vi "Acquisition.vi"() -> ()   [LabVIEW 2012]
uses:
  Type/_Run State.ctl
  Type/_File Type.ctl
  Type/_RT Command.ctl
  Type/_Data Operation.ctl
  Type/_Run Module.ctl
  Configuration/_Global Configuration.vi
  <vilib>/Utility/config.llb/Read Key (Path).vi
  <vilib>/Utility/config.llb/Read Key (String).vi
  <vilib>/Utility/config.llb/Write Key (Path).vi
  <vilib>/Utility/config.llb/Write Key (String).vi
  <vilib>/Utility/file.llb/Read From Spreadsheet File (string).vi
  <vilib>/Utility/config.llb/NI_LVConfig.lvlib
  <vilib>/Utility/miscctls.llb/LVRectTypeDef.ctl
panel:
  in  "Equilibration Time":u32
  in  "Editor":bool
  out "# of Samp":i32=1 caption="# of Samples"
  in  "Sample Description":string
  in  "Sync Mode":enum32{"Manual", "LC Sync"}(radio)
  in  "Data Folder":path
  in  "Save":bool
  in  "Load":bool
  in  "Insert":bool
  in  "Delete":bool
  in  "Import":bool
  in  "Export":bool
  in  "Sample List":i32(listbox)
  in  "Run":bool
  in  "Cancel":bool
  in  "List File":path
  out "Run Time":i32=1 caption="Run Time (ms)"
  in  "Current Sample":i32=1 min=0
  in  "Method File":path
  # "(mS)"
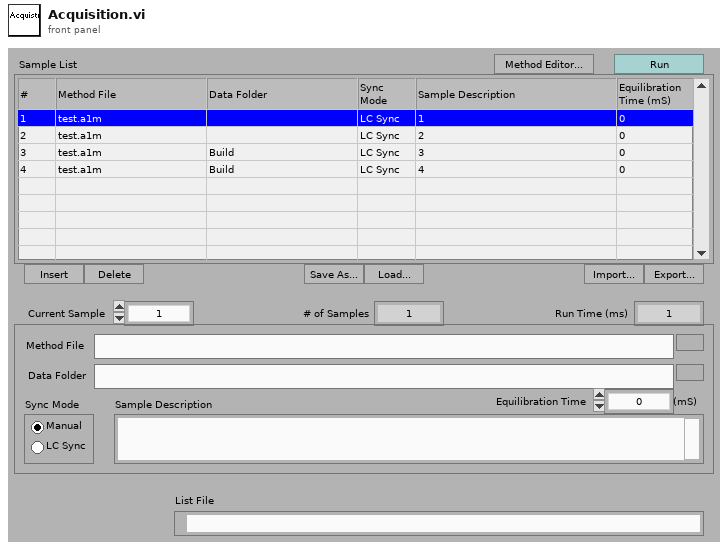
[diagram p1: front panel]
types:
  T1 = typedef "_Run State.ctl" = enum16{"Init", "Update", "Start", "End", "Error"}
  T2 = typedef "_File Type.ctl" = enum16{"Configuration", "Old Configuration", "Calibration", "Resolution", "Diagnostic Method", "Old Method", "Acq Method", "Samp List"}
  T3 = typedef "LVRectTypeDef.ctl" = cluster{"Left":i16, "Top":i16, "Right":i16, "Bottom":i16}
  T4 = typedef "_RT Command.ctl" = enum16{"Start", "Stop", "Runtime Update", "Get Data", "Get Info", "Get Status", "Get Param", "Get Config", "Get Table", "Read ADC", "Set Oscillator", "Update Config", "Update Table", "Set All Pol", "Set Pol and DC", "Set Max Mass", "Toggle RP", "Toggle EL", "Set PIC", "Initialize Turbo", "Send Turbo Comm", "Close Turbo", "P1", "P2", "P3", "Send Serial", "Set LC Out", "Get LC In", "Read VAC", "Test Table", "Toggle Power", "Get Startup", "Set Startup", "Get ADC Table", "Set ADC Table", "Get Brief Status", "Get Detail Status", "Auxiliary Update", "Set CC Logics", "Set CC Input Logics", "Ignore Error"}
  T5 = typedef "_Data Operation.ctl" = enum8{"Initialize", "Get Data", "Set Data", "Close"}
  T6 = enum32{"Bad", "Idle", "Run top level", "Running"}
  T7 = enum32{"existing file", "new file", "new or existing file", "existing dir", "new dir", "new or existing dir", "existing file (use LLBs)", "new file (use LLBs)", "new or existing file (use LLBs)", "new or existing file or directory (use LLBs)"}
  T8 = typedef "NI_LVConfig.lvlib/Config Data RefNum.ctl" = refnum<k1>
  T9 = cluster{"Update":bool, "Running":bool, "List File":path, "Sample List":string[][]}
  T10 = typedef "_Run Module.ctl" = u16
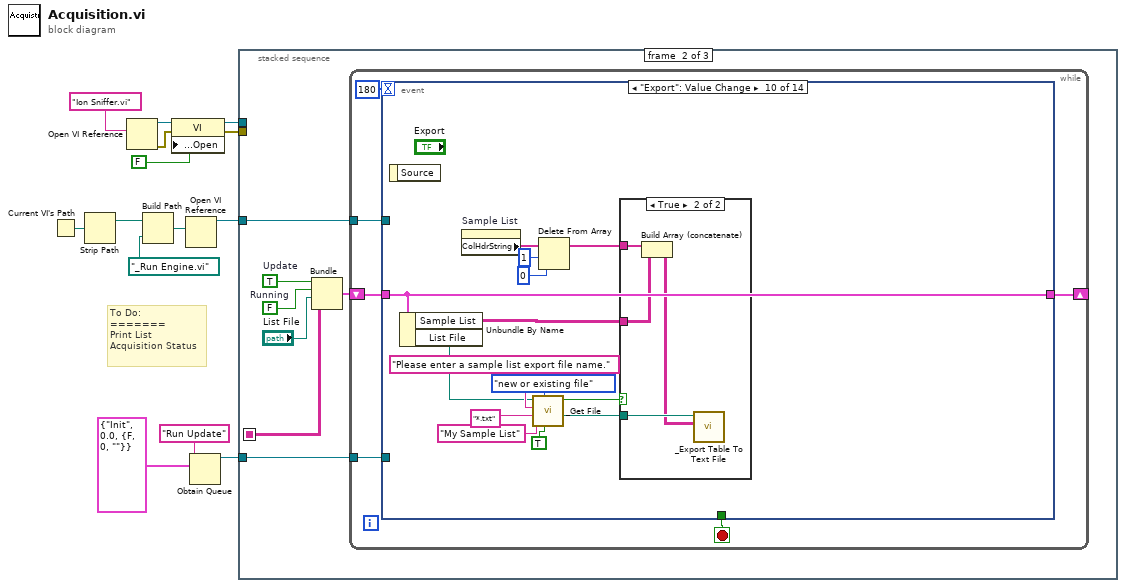
[diagram p0: block diagram]
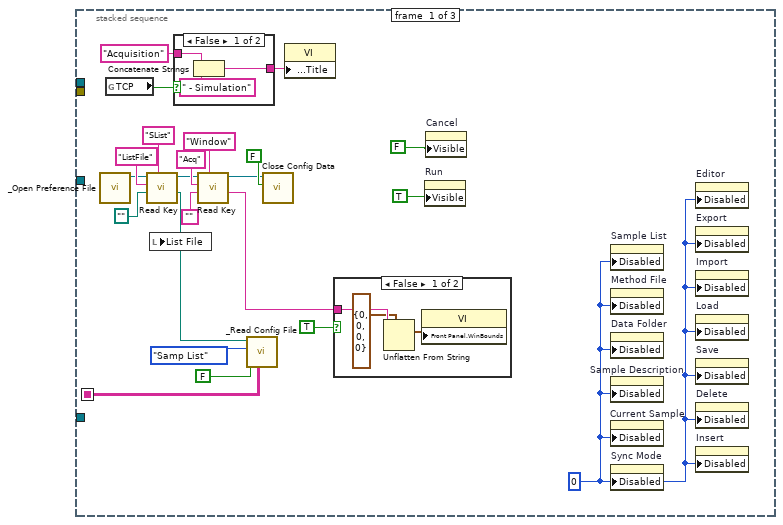
[diagram p2: hidden frame]
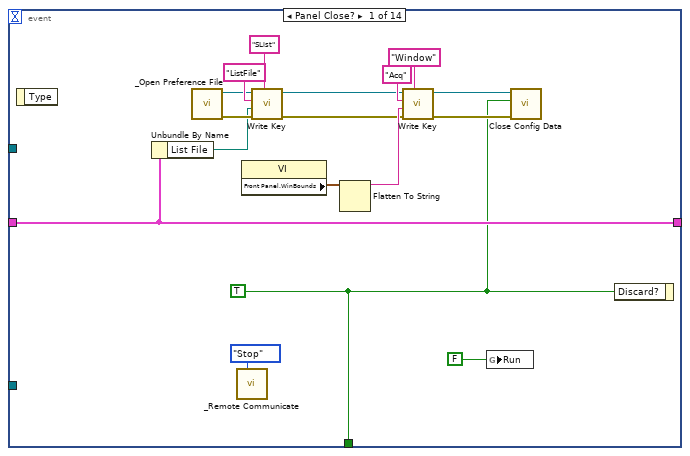
[diagram p5: hidden frame]
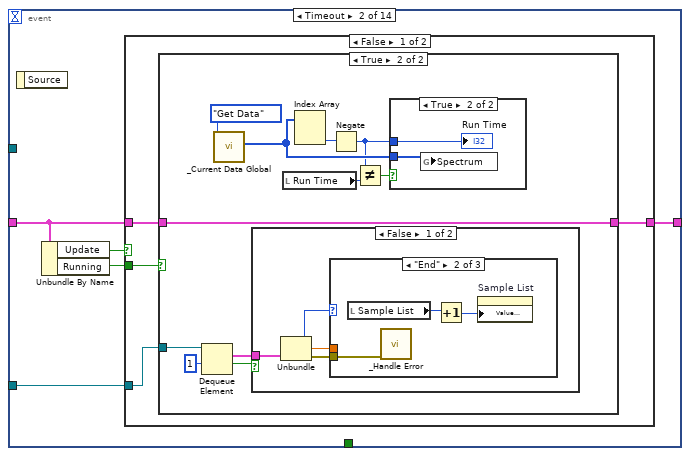
[diagram p6: hidden frame]
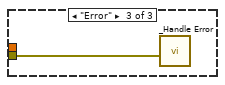
[diagram p10: hidden frame]
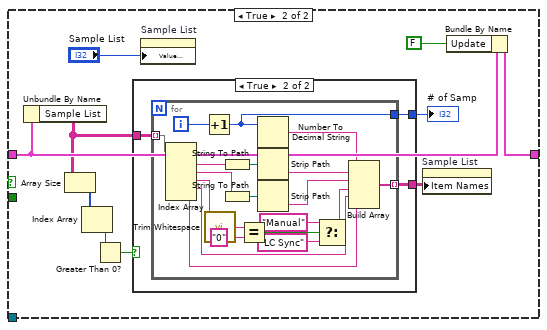
[diagram p12: hidden frame]
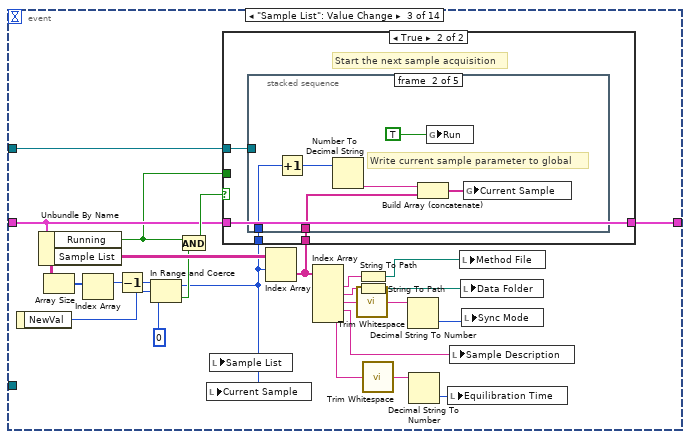
[diagram p14: hidden frame]
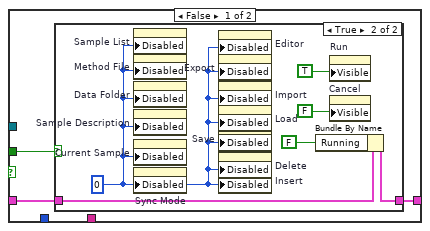
[diagram p15: hidden frame]
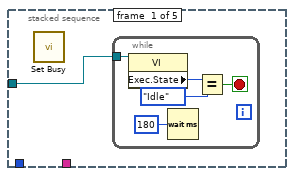
[diagram p17: hidden frame]
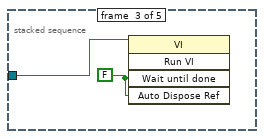
[diagram p18: hidden frame]
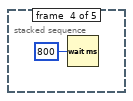
[diagram p19: hidden frame]
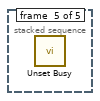
[diagram p20: hidden frame]
diagram:
  # "To Do:\n=======\nPrint List\nAcquisition Status"
  n1 = Current VI's Path() -> (path=w11:path)
  n2 = Strip Path(path=w11) -> (stripped path=w7:path)  [unwired: 1 out]
  n3 = Open VI Reference(vi path="Ion Sniffer.vi") -> (vi reference=w5:refnum<vi>, error out=w4:errorcluster)  [unwired: 1 in, 4 out]
  n4 = Build Path(base path=w7, name or relative path=path "_Run Engine.vi") -> (appended path=w9:path)
  n5 = property class="VI"(reference=w5, error in=w4, "Front Panel Window:Open"=FALSE) -> (reference out=w2:refnum<vi>, error out=w1:errorcluster)
  n6 = Open VI Reference(vi path=w9) -> (vi reference=w8:refnum<vi>)  [unwired: 1 in, 5 out]
  n7 = Obtain Queue(name (unnamed)="Run Update", element data type=cluster{T1, dbl, "error out":errorcluster} {enum."Init", 0.0, "error out"={"status"=FALSE, "code"=0, "source"=""}}) -> (queue out=w12:refnum<queue>)  [unwired: 3 in, 2 out]
  n8 = stacked-sequence {
    seq-local: [w17 _ _] -> [_ w44 _]
    tunnel: w12 -> [_ w50 w346]
    tunnel: w8 -> [_ w49 w345]
    tunnel: w2 -> [_ _ w341]
    tunnel: w1 -> [_ _ w340]
    frame #0 {
      w16 = u8 0 ("Disabled")
      n9 = call "_Open Preference File.vi"() -> ("refnum"=w22:T8)  [unwired: 1 in, 6 out]
      n10 = global read "_Global Configuration.vi" "TCP"() -> (w34:bool)
      n11 = call-poly <vilib>:"Read Key.vi"("section"="SList", "default value"=path "", "key"="ListFile", "refnum"=w22) -> ("value"=w18:path, "refnum out"=w23:T8)  [unwired: 1 in, 5 out]
      n12 = local write "List File"(w18) -> ()
      n13 = case shown="False" w34 {
        tunnel: "Acquisition" ("string") -> [w42 w43]
        tunnel: [w40 w43] -> w35
        frame False {
          n14 = Concatenate Strings(w42, " - Simulation" ("string")) -> (w40:string)
        }
        frame True {
        }
      }
      n15 = call-poly <vilib>:"Read Key.vi"("section"="Window", "default value"="", "key"="Acq" ("section"), "refnum"=w23) -> ("value"=w25:string, "refnum out"=w21:T8)  [unwired: 2 in, 4 out]
      n16 = call "_Read Config File.vi"("advisory dialog? (display:T)"=FALSE, "File Type (config)"=_File_Type."Samp List", "start path  (Not A Path)"=w18) -> ("Sample List"=w17:string[][])  [unwired: 8 out]
      n17 = call <vilib>:"Close Config Data.vi"("write file if changed (T)"=FALSE ("write configuration file? (F)"), "refnum"=w21) -> ()  [unwired: 1 in, 9 out]
      n18 = property class="VI"("Front Panel Window:Title"=w35) -> ()  [unwired: 2 in, 2 out]
      n19 = case shown="False" TRUE {
        tunnel: w25 -> [w39 _]
        frame False {
          n20 = Unflatten From String(type=T3 {"Left"=0, "Top"=0, "Right"=0, "Bottom"=0} ("Front Panel Window:Window Bounds"), binary string=w39) -> (value=w37:T3)  [unwired: 1 in, 4 out]
          n21 = property class="VI"("Front Panel.WinBounds"=w37) -> ()  [unwired: 2 in, 2 out]
        }
        frame True {
        }
      }
      n22 = property on="Run" class="Bool"("Visible"=TRUE) -> ()  [unwired: 2 in, 2 out]
      n23 = property on="Cancel" class="Bool"("Visible"=FALSE ("Unit")) -> ()  [unwired: 2 in, 2 out]
      n24 = property on="Sample List" class="MCListbox (strict)"("Disabled"=w16) -> ()  [unwired: 2 in, 2 out]
      n25 = property on="Method File" class="Path"("Disabled"=w16) -> ()  [unwired: 2 in, 2 out]
      n26 = property on="Data Folder" class="Path"("Disabled"=w16) -> ()  [unwired: 2 in, 2 out]
      n27 = property on="Sample Description" class="Str"("Disabled"=w16) -> ()  [unwired: 2 in, 2 out]
      n28 = property on="Current Sample" class="DigNum (strict)"("Disabled"=w16) -> ()  [unwired: 2 in, 2 out]
      n29 = property on="Sync Mode" class="RadioBtnsControl (strict)"("Disabled"=w16) -> ()  [unwired: 2 in, 2 out]
      n30 = property on="Editor" class="Bool"("Disabled"=w16) -> ()  [unwired: 2 in, 2 out]
      n31 = property on="Export" class="Bool"("Disabled"=w16) -> ()  [unwired: 2 in, 2 out]
      n32 = property on="Import" class="Bool"("Disabled"=w16) -> ()  [unwired: 2 in, 2 out]
      n33 = property on="Load" class="Bool"("Disabled"=w16) -> ()  [unwired: 2 in, 2 out]
      n34 = property on="Save" class="Bool"("Disabled"=w16) -> ()  [unwired: 2 in, 2 out]
      n35 = property on="Delete" class="Bool"("Disabled"=w16) -> ()  [unwired: 2 in, 2 out]
      n36 = property on="Insert" class="Bool"("Disabled"=w16) -> ()  [unwired: 2 in, 2 out]
    }
    frame #1 {
      w47 = FALSE  # Running
      w48 = TRUE  # Update
      n37 = Bundle("Update"=w48, "Running"=w47, "List File"="List File", "Sample List"=w44) -> (w46:T9)  [unwired: 1 out]
      n38 = while {
        shift-right: [w53] -> _
        shift-left: w46 -> [w55]
        tunnel: w50 -> [w52]
        tunnel: w49 -> [w51]
        stop <- w56 stop-if-true
        n39 = event shown="[9] \"Export\": Value Change" {
          selector: _ -> [_ _ _ _ _ _ _ _ _ _ _ _ _ _]
          dyn-events: _ -> [_ _ _ _ _ _ _ _ _ _ _ _ _ _]
          timeout: 180 -> [_ _ _ _ _ _ _ _ _ _ _ _ _ _]
          tunnel: [w57 _ _ _ _ _ _ _ _ _ _ _ _ _] -> w56
          tunnel: w55 -> [w68 w76 w145 w193 w209 w222 w230 w244 w252 w272 w308 w311 w325 w339]
          tunnel: [w68 w78 w144 w193 w208 w220 w228 w242 w251 w272 w310 w318 w321 w339] -> w53
          tunnel: w52 -> [_ w77 _ _ _ _ _ _ _ _ _ w320 _ _]
          tunnel: w51 -> [_ _ w146 _ _ _ _ _ _ _ _ _ w324 _]
          event Panel Close? {
            w57 = TRUE ("Discard?")
            n40 = event-data() -> ()  [unwired: 2 out]
            n41 = Unbundle By Name(w68) -> ("List File"=w67:path)
            n42 = call "_Open Preference File.vi"() -> ("error"=w70:errorcluster, "refnum"=w71:T8)  [unwired: 1 in, 5 out]
            n43 = call "_Remote Communicate.vi"("Command"=_RT_Command."Stop") -> ()  [unwired: 5 in, 4 out]
            n44 = property class="VI"() -> ("Front Panel.WinBounds"=w65:T3)  [unwired: 2 in, 2 out]
            n45 = call-poly <vilib>:"Write Key.vi"("section"="SList", "error in (no error)"=w70, "value"=w67, "key"="ListFile", "refnum"=w71) -> ("error out"=w58:errorcluster, "refnum out"=w59:T8)  [unwired: 5 out]
            n46 = Flatten To String(anything=w65) -> (data string=w64:string)  [unwired: 1 in, 4 out]
            n47 = call-poly <vilib>:"Write Key.vi"("section"="Window", "error in (no error)"=w58, "value"=w64, "key"="Acq" ("section"), "refnum"=w59) -> ("error out"=w60:errorcluster, "refnum out"=w61:T8)  [unwired: 1 in, 4 out]
            n48 = global write "_Global Configuration.vi" "Run"(FALSE ("Update")) -> ()
            n49 = call <vilib>:"Close Config Data.vi"("error in (no error)"=w60, "write file if changed (T)"=w57, "refnum"=w61) -> ()  [unwired: 9 out]
            n50 = event-data("Discard?"=w57) -> ()  [unwired: 1 in, 1 out]
          }
          event Timeout {
            n51 = event-data() -> ()  [unwired: 2 out]
            n52 = Unbundle By Name(w76) -> ("Update"=w75:bool, "Running"=w74:bool)
            n53 = case shown="False" w75 {
              tunnel: w76 -> [w80 w114]
              tunnel: [w79 w112] -> w78
              tunnel: w74 -> [w82 _]
              tunnel: w77 -> [w81 _]
              frame False {
                n54 = case shown="True" w82 {
                  tunnel: w81 -> [_ w94]
                  tunnel: w80 -> [w83 w84]
                  tunnel: [w83 w84] -> w79
                  frame False {
                  }
                  frame True {
                    n55 = Dequeue Element(queue=w94, timeout in ms (-1)=1) -> (element=w92:cluster{T1, dbl, "error out":errorcluster}, timed out?=w91:bool)  [unwired: 1 in, 2 out]
                    n56 = call "_Current Data Global.vi"("Operation"=_Data_Operation."Get Data") -> ("Latest Raw Data"=w87:i32[])  [unwired: 3 in, 3 out]
                    n57 = case shown="False" w91 {
                      tunnel: w92 -> [w100 _]
                      frame False {
                        n58 = Unbundle(w100) -> (w99:T1, w97:dbl, "error out"=w98:errorcluster)
                        n59 = case shown="\"End\"" w99 {
                          tunnel: w98 -> [_ w103 w104]
                          tunnel: w97 -> [_ _ _]
                          frame "Init", Default {
                          }
                          frame "End" {
                            n60 = local read "Sample List"() -> (w102:i32)
                            n61 = call "_Handle Error.vi"("error in (no error)"=w103) -> ()  [unwired: 2 in, 5 out]
                            n62 = Increment(x=w102) -> (x+1=w101:i32)
                            n63 = property on="Sample List" class="MCListbox (strict)"("Value (Signaling)"=w101) -> ()  [unwired: 2 in, 2 out]
                          }
                          frame "Error" {
                            n64 = call "_Handle Error.vi"("error in (no error)"=w104) -> ()  [unwired: 2 in, 5 out]
                          }
                        }
                      }
                      frame True {
                      }
                    }
                    n65 = local read "Run Time"() -> (w89:i32)
                    n66 = Index Array(array=w87) -> (element #2=w86:i32)  [unwired: 2 in, 1 out]
                    n67 = Negate(x=w86) -> (-x=w85:i32)
                    n68 = Not Equal?(x=w85, y=w89) -> (x != y?=w88:bool)
                    n69 = case shown="True" w88 {
                      tunnel: w87 -> [_ w95]
                      tunnel: w85 -> [_ w96]
                      frame False {
                      }
                      frame True {
                        n70 = global write "_Global Configuration.vi" "Spectrum"(w95) -> ()
                        "Run Time" <- w96
                      }
                    }
                  }
                }
              }
              frame True {
                n71 = Unbundle By Name(w114) -> ("Sample List"=w108:string[][])
                n72 = Array Size(array=w108) -> (size(s)=w107:i32[])
                n73 = Index Array(array=w107) -> (element=w106:i32)  [unwired: 1 in]
                n74 = Greater Than 0?(x=w106) -> (x > 0?=w105:bool)
                n75 = case shown="True" w105 {
                  tunnel: [_ w117] -> w110
                  tunnel: [_ w116] -> w109
                  tunnel: w108 -> [_ w115]
                  frame False {
                  }
                  frame True {
                    n76 = for {
                      tunnel: w115 -> [w137] mode=indexing
                      tunnel: [w135] -> w117
                      tunnel: [w120] -> w116 mode=indexing
                      i -> [w136]
                      n77 = Index Array(array=w137) -> (element #1=w134:string, element #2=w131:string, element #3=w130:string, element #4=w121:string, element #5=w118:string)  [unwired: 5 in]
                      n78 = Increment(x=w136) -> (x+1=w135:i32)
                      n79 = call <vilib>:"Trim Whitespace.vi"("string"=w130) -> ("trimmed string"=w128:string)  [unwired: 1 in]
                      n80 = String To Path(string=w134) -> (path=w133:path)
                      n81 = String To Path(string=w131) -> (path=w132:path)
                      n82 = Equal?(x=w128, y="0") -> (x = y?=w129:bool)
                      n83 = Number To Decimal String(number=w135) -> (decimal integer string=w125:string)  [unwired: 1 out]
                      n84 = Strip Path(path=w133) -> (name=w124:string)  [unwired: 1 out]
                      n85 = Strip Path(path=w132) -> (name=w123:string)  [unwired: 1 out]
                      n86 = Select(t="Manual" ("y"), s=w129, f="LC Sync" ("y")) -> (s? t:f=w122:string)
                      n87 = Build Array(w125, w124, w123, w122, w121, w118) -> (w120:string[])
                    }
                  }
                }
                "# of Samp" <- w110
                n88 = property on="Sample List" class="MCListbox (strict)"("Value (Signaling)"="Sample List") -> ()  [unwired: 2 in, 2 out]
                n89 = property on="Sample List" class="MCListbox (strict)"("Item Names"=w109) -> ()  [unwired: 2 in, 2 out]
                n90 = Bundle By Name(cluster=w114, "Update"=FALSE) -> (w112:T9)
              }
            }
          }
          event "Sample List": Value Change {
            n91 = event-data() -> ("NewVal"=w162:i32)  [unwired: 1 out]
            n92 = Unbundle By Name(w145) -> ("Running"=w143:bool, "Sample List"=w159:string[][])
            n93 = Array Size(array=w159) -> (size(s)=w157:i32[])
            n94 = Index Array(array=w157) -> (element=w158:i32)  [unwired: 1 in]
            n95 = Decrement(x=w158) -> (x-1=w160:i32)
            n96 = In Range and Coerce(upper limit=w160, x=w162, lower limit=0) -> (coerced(x)=w141:i32, In Range?=w148:bool)
            n97 = And(x=w143, y=w148) -> (x .and. y?=w147:bool)
            n98 = local write "Current Sample"(w141) -> ()
            n99 = local write "Sample List"(w141) -> ()
            n100 = Index Array(array=w159, index (row)=w141) -> (element=w142:string[])  [unwired: 1 in]
            n101 = case shown="True" w147 {
              tunnel: w146 -> [_ w176]
              tunnel: w145 -> [w165 w175]
              tunnel: [w164 w175] -> w144
              tunnel: w143 -> [w163 _]
              tunnel: w142 -> [_ w174]
              tunnel: w141 -> [_ w173]
              frame False {
                n102 = case shown="True" w163 {
                  tunnel: w165 -> [w166 w172]
                  tunnel: [w166 w171] -> w164
                  frame False {
                  }
                  frame True {
                    w170 = u8 0 ("Disabled")
                    n103 = property on="Sample List" class="MCListbox (strict)"("Disabled"=w170) -> ()  [unwired: 2 in, 2 out]
                    n104 = property on="Method File" class="Path"("Disabled"=w170) -> ()  [unwired: 2 in, 2 out]
                    n105 = property on="Data Folder" class="Path"("Disabled"=w170) -> ()  [unwired: 2 in, 2 out]
                    n106 = property on="Sample Description" class="Str"("Disabled"=w170) -> ()  [unwired: 2 in, 2 out]
                    n107 = property on="Current Sample" class="DigNum (strict)"("Disabled"=w170) -> ()  [unwired: 2 in, 2 out]
                    n108 = property on="Sync Mode" class="RadioBtnsControl (strict)"("Disabled"=w170) -> ()  [unwired: 2 in, 2 out]
                    n109 = property on="Editor" class="Bool"("Disabled"=w170) -> ()  [unwired: 2 in, 2 out]
                    n110 = property on="Export" class="Bool"("Disabled"=w170) -> ()  [unwired: 2 in, 2 out]
                    n111 = property on="Import" class="Bool"("Disabled"=w170) -> ()  [unwired: 2 in, 2 out]
                    n112 = property on="Load" class="Bool"("Disabled"=w170) -> ()  [unwired: 2 in, 2 out]
                    n113 = property on="Save" class="Bool"("Disabled"=w170) -> ()  [unwired: 2 in, 2 out]
                    n114 = property on="Delete" class="Bool"("Disabled"=w170) -> ()  [unwired: 2 in, 2 out]
                    n115 = property on="Insert" class="Bool"("Disabled"=w170) -> ()  [unwired: 2 in, 2 out]
                    n116 = Bundle By Name(cluster=w172, "Running"=FALSE) -> (w171:T9)
                    n117 = property on="Run" class="Bool"("Visible"=TRUE) -> ()  [unwired: 2 in, 2 out]
                    n118 = property on="Cancel" class="Bool"("Visible"=FALSE) -> ()  [unwired: 2 in, 2 out]
                  }
                }
              }
              frame True {
                # "Start the next sample acquisition"
                n119 = stacked-sequence {
                  tunnel: w176 -> [w177 _ w189 _ _]
                  tunnel: w174 -> [_ w187 _ _ _]
                  tunnel: w173 -> [_ w184 _ _ _]
                  frame #0 {
                    n120 = call <vilib>:"Set Busy.vi"() -> ()  [unwired: 4 in, 8 out]
                    n121 = while {
                      tunnel: w177 -> [w182]
                      stop <- w179 stop-if-true
                      n122 = property class="VI"(reference=w182) -> ("Exec.State"=w181:T6)  [unwired: 1 in, 2 out]
                      n123 = Wait (ms)(milliseconds to wait=u32 180) -> ()  [unwired: 1 out]
                      n124 = Equal?(x=w181, y=T6."Idle") -> (x = y?=w179:bool)
                    }
                  }
                  frame #1 {
                    # "Write current sample parameter to global"
                    n125 = Increment(x=w184) -> (x+1=w183:i32)
                    n126 = Number To Decimal String(number=w183) -> (decimal integer string=w185:string)  [unwired: 1 out]
                    n127 = Build Array (concatenate)(w185, w187) -> (w186:string[])
                    n128 = global write "_Global Configuration.vi" "Run"(TRUE ("Update")) -> ()
                    n129 = global write "_Global Configuration.vi" "Current Sample"(w186) -> ()
                  }
                  frame #2 {
                    w190 = FALSE ("Wait until done")
                    n130 = invoke class="VI" method="Run VI"(reference=w189, "Wait until done"=w190, "Auto Dispose Ref"=w190) -> ()  [unwired: 2 in, 5 out]
                  }
                  frame #3 {
                    n131 = Wait (ms)(milliseconds to wait=u32 800) -> ()  [unwired: 1 out]
                  }
                  frame #4 {
                    n132 = call <vilib>:"Unset Busy.vi"() -> ()  [unwired: 2 in, 10 out]
                  }
                }
              }
            }
            n133 = Index Array(array=w142) -> (element #1=w153:string, element #2=w154:string, element #3=w155:string, element #4=w156:string, element #5=w139:string)  [unwired: 5 in]
            n134 = call <vilib>:"Trim Whitespace.vi"("string"=w155) -> ("trimmed string"=w150:string)  [unwired: 1 in]
            n135 = String To Path(string=w153) -> (path=w152:path)
            n136 = String To Path(string=w154) -> (path=w151:path)
            n137 = call <vilib>:"Trim Whitespace.vi"("string"=w139) -> ("trimmed string"=w140:string)  [unwired: 1 in]
            n138 = Decimal String To Number(string=w150) -> (number=w149:i32)  [unwired: 3 out]
            n139 = Decimal String To Number(string=w140) -> (number=w138:i32)  [unwired: 3 out]
            n140 = local write "Equilibration Time"(w138) -> ()
            n141 = local write "Sample Description"(w156) -> ()
            n142 = local write "Method File"(w152) -> ()
            n143 = local write "Data Folder"(w151) -> ()
            n144 = local write "Sync Mode"(w149) -> ()
          }
          event "Current Sample": Value Change {
            n145 = event-data() -> ("NewVal"=w192:i32)  [unwired: 1 out]
            n146 = property on="Sample List" class="MCListbox (strict)"("Value (Signaling)"=w192) -> ()  [unwired: 2 in, 2 out]
          }
          event "Insert": Value Change {
            n147 = event-data() -> ()  [unwired: 2 out]
            n148 = call "Please enter # of samples to insert."() -> ("# of Samples to Insert"=w206:dbl)  [unwired: 2 in, 17 out]
            n149 = Unbundle By Name(w209) -> ("Sample List"=w201:string[][])
            n150 = local read "Sample List"() -> (w200:i32)
            n151 = To Long Integer(number=w206) -> (32bit integer=w205:i32)
            n152 = In Range and Coerce(upper limit=2147483647, x=w205, lower limit=1) -> (coerced(x)=w202:i32)  [unwired: 1 out]
            n153 = Index Array(array=w201, index (row)=w200) -> (element=w196:string[])  [unwired: 1 in]
            n154 = Array Size(array=w196) -> (size(s)=w198:i32)
            n155 = Greater Than 0?(x=w198) -> (x > 0?=w197:bool)
            n156 = Select(t=w196, s=w197, f=string[] ["", "", "1", "", "0"] ("appended array")) -> (s? t:f=w194:string[])
            n157 = for {
              N: w202 -> [_]
              shift-right: [w211] -> w199
              shift-left: w201 -> [w213]
              tunnel: w200 -> [w212]
              tunnel: w194 -> [w210]
              n158 = Insert Into Array(array=w213, index (row)=w212, new element=w210) -> (w211:string[][])  [unwired: 1 in]
            }
            n159 = Bundle By Name(cluster=w209, "Sample List"=w199, "Update"=TRUE) -> (w208:T9)
          }
          event "Delete": Value Change {
            n160 = event-data() -> ()  [unwired: 2 out]
            n161 = Unbundle By Name(w222) -> ("Sample List"=w221:string[][])
            n162 = Two Button Dialog(message="Please choose a delete option.", 1:"Delete All Samples" ("T button name (\"OK\")"), 2:"Delete Current Sample" ("T button name (\"OK\")")) -> (T button?=w214:bool)
            n163 = case shown="True" w214 {
              tunnel: w221 -> [_ w226]
              tunnel: [_ w223] -> w219
              frame False {
              }
              frame True {
                n164 = local read "Sample List"() -> (w224:i32)
                n165 = Delete From Array(array=w226, length=1, index (row)=w224) -> (array with subset deleted=w223:string[][])  [unwired: 1 in, 1 out]
              }
            }
            n166 = Bundle By Name(cluster=w222, "Sample List"=w219, "Update"=TRUE) -> (w220:T9)
          }
          event "Save": Value Change {
            n167 = event-data() -> ()  [unwired: 2 out]
            n168 = Unbundle By Name(w230) -> ("List File"=w232:path, "Sample List"=w231:string[][])
            n169 = call "_Save Config File.vi"("Sample List"=w231, "File Type (config)"=_File_Type."Samp List", "start path  (Not A Path)"=w232) -> ("error"=w229:bool, "new file path"=w227:path)  [unwired: 5 in, 2 out]
            n170 = case shown="False" w229 {
              tunnel: w230 -> [w236 w237]
              tunnel: [w235 w237] -> w228
              tunnel: w227 -> [w234 _]
              frame False {
                n171 = local write "List File"(w234) -> ()
                n172 = Bundle By Name(cluster=w236, "List File"=w234) -> (w235:T9)
              }
              frame True {
              }
            }
          }
          event "Load": Value Change {
            n173 = event-data() -> ()  [unwired: 2 out]
            n174 = Unbundle By Name(w244) -> ("List File"=w241:path)
            n175 = call "_Read Config File.vi"("File Type (config)"=_File_Type."Samp List", "start path  (Not A Path)"=w241) -> ("error"=w243:bool, "new file path"=w238:path, "Sample List"=w239:string[][])  [unwired: 3 in, 4 out]
            n176 = case shown="False" w243 {
              tunnel: w244 -> [w249 w250]
              tunnel: [w248 w250] -> w242
              tunnel: w238 -> [w247 _]
              tunnel: w239 -> [w245 _]
              frame False {
                n177 = Bundle By Name(cluster=w249, "Update"=TRUE, "Sample List"=w245, "List File"=w247) -> (w248:T9)
                n178 = local write "List File"(w247) -> ()
              }
              frame True {
              }
            }
          }
          event "Import": Value Change {
            n179 = event-data() -> ()  [unwired: 2 out]
            n180 = Unbundle By Name(w252) -> ("List File"=w255:path)
            n181 = call "_Get File.vi"("For Write (T)"=FALSE, "select mode (new or existing)"=T7."existing file", "extension (isd)"="*.txt" ("pattern (all files)"), "prompt"="Please select a sample list import file.", "Start Path"=w255) -> ("Seleted File"=w253:path, "Exists"=w261:bool, "Succeeded"=w260:bool)  [unwired: 1 in, 1 out]
            n182 = And(x=w260, y=w261) -> (x .and. y?=w254:bool)
            n183 = case shown="True" w254 {
              tunnel: w253 -> [_ w267]
              tunnel: w252 -> [w262 w266]
              tunnel: [w262 w265] -> w251
              frame False {
              }
              frame True {
                n184 = call-poly <vilib>:"Read From Spreadsheet File.vi"("file path (dialog if empty)"=w267) -> ("all rows"=w269:string[][])  [unwired: 3 in, 7 out]
                n185 = Delete From Array(array=w269, length=1, index (row)=0) -> (array with subset deleted=w264:string[][])  [unwired: 1 in, 1 out]
                n186 = Bundle By Name(cluster=w266, "Update"=TRUE, "Sample List"=w264) -> (w265:T9)
              }
            }
          }
          event "Export": Value Change {
            n187 = event-data() -> ()  [unwired: 2 out]
            n188 = Unbundle By Name(w272) -> ("Sample List"=w273:string[][], "List File"=w280:path)
            n189 = property on="Sample List" class="MCListbox (strict)"() -> ("ColHdrString"=w277:string[])  [unwired: 2 in, 2 out]
            n190 = call "_Get File.vi"("For Write (T)"=TRUE, "select mode (new or existing)"=T7."new or existing file", "default name"="My Sample List", "extension (isd)"="*.txt" ("pattern (all files)"), "prompt"="Please enter a sample list export file name.", "Start Path"=w280) -> ("Seleted File"=w279:path, "Succeeded"=w278:bool)  [unwired: 2 out]
            n191 = Delete From Array(array=w277, length=1, index=0) -> (array with subset deleted=w274:string[])  [unwired: 1 out]
            n192 = case shown="True" w278 {
              tunnel: w279 -> [_ w286]
              tunnel: w274 -> [_ w288]
              tunnel: w273 -> [_ w287]
              frame False {
              }
              frame True {
                n193 = Build Array (concatenate)(w288, w287) -> (w285:string[][])
                n194 = call "_Export Table To Text File.vi"("2D data"=w285, "file path (dialog if empty)"=w286) -> ()  [unwired: 4 in, 3 out]
              }
            }
          }
          event "Method File", "Data Folder", "Sync Mode", "Sample Description", "Equilibration Time": Value Change {
            n195 = event-data() -> ()  [unwired: 2 out]
            n196 = Unbundle By Name(w308) -> ("Sample List"=w296:string[][])
            n197 = Path To String(path="Data Folder") -> (string=w304:string)
            n198 = Path To String(path="Method File") -> (string=w305:string)
            n199 = Index Array(array=w296, index (row)=0) -> (element=w299:string[])  [unwired: 1 in]
            n200 = Number To Decimal String(number="Sync Mode") -> (decimal integer string=w301:string)  [unwired: 1 out]
            n201 = Number To Decimal String(number="Equilibration Time") -> (decimal integer string=w289:string)  [unwired: 1 out]
            n202 = Array Size(array=w299) -> (size(s)=w298:i32)
            n203 = Build Array(w305, w304, w301, "Sample Description", w289) -> (w294:string[])
            n204 = Greater Than 0?(x=w298) -> (x > 0?=w297:bool)
            n205 = Replace Array Subset(array=w296, new element=w294, index (row)="Current Sample") -> (w292:string[][])  [unwired: 1 in]
            n206 = Insert Into Array(array=w296, index (row)="Current Sample", new element=w294) -> (w293:string[][])  [unwired: 1 in]
            n207 = Select(t=w292, s=w297, f=w293) -> (s? t:f=w291:string[][])
            n208 = Bundle By Name(cluster=w308, "Update"=TRUE, "Sample List"=w291) -> (w310:T9)
          }
          event "Run": Value Change {
            w315 = T10 2 items=["Diagnostics", "Tune", "Acquisition"] ("RunModule")
            w314 = u8 1 ("Disabled")
            n209 = event-data() -> ()  [unwired: 2 out]
            n210 = Flush Queue(queue=w320) -> ()  [unwired: 1 in, 3 out]
            n211 = global write "_Global Configuration.vi" "RunModule"(w315) -> ()
            n212 = property on="Sample List" class="MCListbox (strict)"("Value (Signaling)"=0) -> ()  [unwired: 2 in, 2 out]
            n213 = property on="Run" class="Bool"("Visible"=FALSE) -> ()  [unwired: 2 in, 2 out]
            n214 = property on="Cancel" class="Bool"("Visible"=TRUE) -> ()  [unwired: 2 in, 2 out]
            n215 = property on="Sample List" class="MCListbox (strict)"("Disabled"=w314) -> ()  [unwired: 2 in, 2 out]
            n216 = property on="Method File" class="Path"("Disabled"=w314) -> ()  [unwired: 2 in, 2 out]
            n217 = property on="Data Folder" class="Path"("Disabled"=w314) -> ()  [unwired: 2 in, 2 out]
            n218 = property on="Sample Description" class="Str"("Disabled"=w314) -> ()  [unwired: 2 in, 2 out]
            n219 = property on="Current Sample" class="DigNum (strict)"("Disabled"=w314) -> ()  [unwired: 2 in, 2 out]
            n220 = property on="Sync Mode" class="RadioBtnsControl (strict)"("Disabled"=w314) -> ()  [unwired: 2 in, 2 out]
            n221 = property on="Editor" class="Bool"("Disabled"=w314) -> ()  [unwired: 2 in, 2 out]
            n222 = property on="Export" class="Bool"("Disabled"=w314) -> ()  [unwired: 2 in, 2 out]
            n223 = property on="Import" class="Bool"("Disabled"=w314) -> ()  [unwired: 2 in, 2 out]
            n224 = property on="Load" class="Bool"("Disabled"=w314) -> ()  [unwired: 2 in, 2 out]
            n225 = property on="Save" class="Bool"("Disabled"=w314) -> ()  [unwired: 2 in, 2 out]
            n226 = property on="Delete" class="Bool"("Disabled"=w314) -> ()  [unwired: 2 in, 2 out]
            n227 = property on="Insert" class="Bool"("Disabled"=w314) -> ()  [unwired: 2 in, 2 out]
            n228 = call "_Launch Dynamic VI.vi"("VI Name"=path "Real Time Display.vi" ("name or relative path")) -> ()  [unwired: 4 out]
            n229 = Bundle By Name(cluster=w311, "Running"=TRUE) -> (w318:T9)
          }
          event "Cancel": Value Change {
            n230 = event-data() -> ()  [unwired: 7 out]
            n231 = stacked-sequence {
              tunnel: w325 -> [_ w328 _]
              tunnel: [_ w328 _] -> w322
              tunnel: w324 -> [_ w327 _]
              frame #0 {
                n232 = call <vilib>:"Set Busy.vi"() -> ()  [unwired: 4 in, 8 out]
                n233 = global write "_Global Configuration.vi" "Run"(FALSE ("Update")) -> ()
              }
              frame #1 {
                n234 = while {
                  tunnel: w327 -> [w333]
                  stop <- w330 stop-if-true
                  n235 = property class="VI"(reference=w333) -> ("Exec.State"=w332:T6)  [unwired: 1 in, 2 out]
                  n236 = Wait (ms)(milliseconds to wait=u32 180) -> ()  [unwired: 1 out]
                  n237 = Equal?(x=w332, y=T6."Idle") -> (x = y?=w330:bool)
                }
              }
              frame #2 {
                w335 = u8 0 ("Disabled")
                n238 = call <vilib>:"Unset Busy.vi"() -> ()  [unwired: 2 in, 10 out]
                n239 = property on="Run" class="Bool"("Visible"=TRUE) -> ()  [unwired: 2 in, 2 out]
                n240 = property on="Cancel" class="Bool"("Visible"=FALSE) -> ()  [unwired: 2 in, 2 out]
                n241 = call "_Remote Wait Until Done.vi"() -> ("error out"=w334:errorcluster)  [unwired: 2 in, 1 out]
                n242 = call "_Remote Park Lens.vi"("error in"=w334) -> ()  [unwired: 1 in, 6 out]
                n243 = property on="Sample List" class="MCListbox (strict)"("Disabled"=w335) -> ()  [unwired: 2 in, 2 out]
                n244 = property on="Method File" class="Path"("Disabled"=w335) -> ()  [unwired: 2 in, 2 out]
                n245 = property on="Data Folder" class="Path"("Disabled"=w335) -> ()  [unwired: 2 in, 2 out]
                n246 = property on="Sample Description" class="Str"("Disabled"=w335) -> ()  [unwired: 2 in, 2 out]
                n247 = property on="Current Sample" class="DigNum (strict)"("Disabled"=w335) -> ()  [unwired: 2 in, 2 out]
                n248 = property on="Sync Mode" class="RadioBtnsControl (strict)"("Disabled"=w335) -> ()  [unwired: 2 in, 2 out]
                n249 = property on="Editor" class="Bool"("Disabled"=w335) -> ()  [unwired: 2 in, 2 out]
                n250 = property on="Export" class="Bool"("Disabled"=w335) -> ()  [unwired: 2 in, 2 out]
                n251 = property on="Import" class="Bool"("Disabled"=w335) -> ()  [unwired: 2 in, 2 out]
                n252 = property on="Load" class="Bool"("Disabled"=w335) -> ()  [unwired: 2 in, 2 out]
                n253 = property on="Save" class="Bool"("Disabled"=w335) -> ()  [unwired: 2 in, 2 out]
                n254 = property on="Delete" class="Bool"("Disabled"=w335) -> ()  [unwired: 2 in, 2 out]
                n255 = property on="Insert" class="Bool"("Disabled"=w335) -> ()  [unwired: 2 in, 2 out]
              }
            }
            n256 = Bundle By Name(cluster=w322, "Running"=FALSE) -> (w321:T9)
          }
          event "Editor": Value Change {
            n257 = event-data() -> ()  [unwired: 2 out]
            n258 = local read "Method File"() -> (w338:path)
            n259 = call "Method Editor.vi"("Method File:"=w338) -> ()
          }
        }
      }
    }
    frame #2 {
      n260 = property class="VI"(reference=w341, error in=w340, "Front Panel Window:Open"=TRUE) -> (reference out=w342:refnum<vi>, error out=w343:errorcluster)
      n261 = Close Reference(reference=w345) -> ()  [unwired: 1 in, 1 out]
      n262 = Release Queue(queue=w346) -> ()  [unwired: 1 in, 4 out]
      n263 = Close Reference(reference=w342, error in (no error)=w343) -> ()  [unwired: 1 out]
    }
  }
